vi "CSUParser.vi"(11 "webpage":string) -> (1 "Time Of Value (s)":dbl format="%#.1f", 2 "RawPressure/mBar":dbl, 3 "status":bool, 4 "MetTimeStamp":timestamp, 5 "ComputerTime":timestamp)   [LabVIEW 2011]
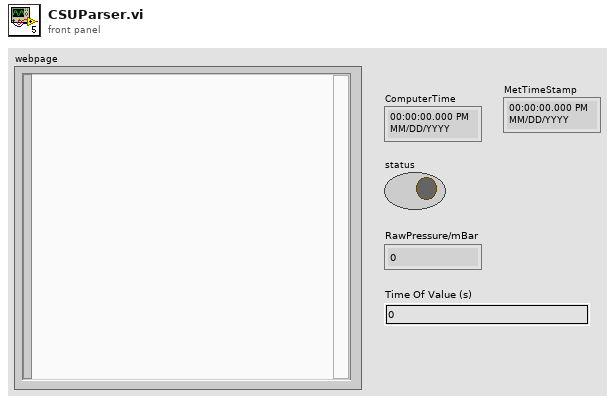
[diagram p1: front panel]
types:
  T1 = cluster{"second":i32, "minute":i32, "hour":i32, "day of month":i32, "month":i32, "year":i32, "day of week":i32, "day of year":i32, "is DST":i32}
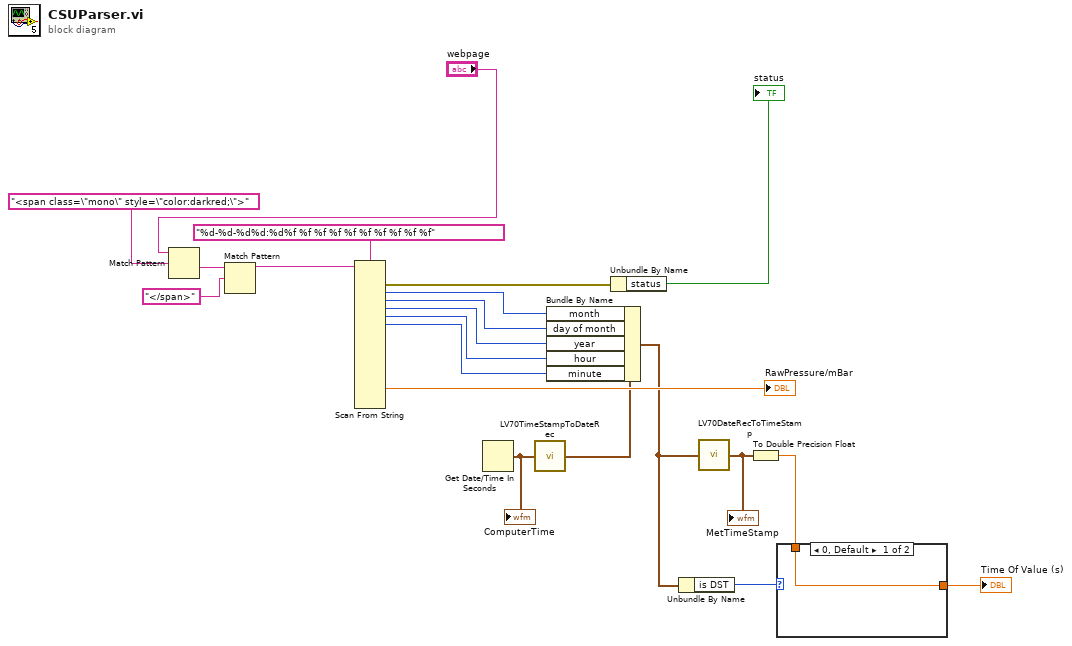
[diagram p0: block diagram]
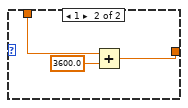
[diagram p2: hidden frame]
diagram:
  n1 = Match Pattern(string="webpage", regular expression="<span class=\"mono\" style=\"color:darkred;\">") -> (after substring=w9:string)  [unwired: 4 out]
  n2 = Match Pattern(string=w9, regular expression="</span>") -> (before substring=w12:string)  [unwired: 4 out]
  n3 = Scan From String(format string="%d-%d-%d%d:%d%f %f %f %f %f %f %f %f %f %f", input string=w12) -> (error out=w15:errorcluster, output 1=w20:i32, output 2=w19:i32, output 3=w18:i32, output 4=w17:i32, output 5=w16:i32, output 13=→"RawPressure/mBar":dbl)  [unwired: 2 in, 26 out]
  n4 = Get Date/Time In Seconds() -> (seconds since 1Jan1904=w7:timestamp)
  "ComputerTime" <- w7
  n5 = call <vilib>:"LV70TimeStampToDateRec.vi"("time stamp"=w7) -> ("date time rec"=w1:T1)
  n6 = Bundle By Name(cluster=w1, "month"=w20, "day of month"=w19, "year"=w18, "hour"=w17, "minute"=w16) -> (w3:T1)
  n7 = Unbundle By Name(w15) -> ("status"=→"status":bool)
  n8 = Unbundle By Name(w3) -> ("is DST"=w4:i32)
  n9 = call <vilib>:"LV70DateRecToTimeStamp.vi"("date time rec"=w3) -> ("Time Stamp"=w2:timestamp)
  "MetTimeStamp" <- w2
  n10 = To Double Precision Float(number=w2) -> (double precision float=w5:dbl)
  n11 = case shown="0, Default" w4 {
    tunnel: w5 -> [w22 w25]
    tunnel: [w22 w23] -> w6
    frame 0, Default {
    }
    frame 1 {
      n12 = Add(x=w25, y=3600.0) -> (x+y=w23:dbl)
    }
  }
  "Time Of Value (s)" <- w6
